vi "Set Version Number.vi"(8 "error in (no error)":errorcluster, 10 "Version number":T1, 11 "NI_AB_API_Targetfile in":refnum<class "NI_AB_API_Build.lvclass">) -> (0 "error out":errorcluster, 3 "NI_AB_API_Targetfile out":refnum<class "NI_AB_API_Build.lvclass">)   [LabVIEW 2020, in "NI_AB_API_Build.lvclass"]
uses:
  <vilib>/AppBuilder/AB_API/Build/NI_AB_API_Build.lvclass
  <vilib>/AppBuilder/AB_API/common/AB_API Version Number.ctl
  <vilib>/AppBuilder/AB_API/Build/NI_AB_API_Build.lvclass/NI_AB_API_Build.ctl
  <vilib>/AppBuilder/AB_Classes/Build/AB_Build.lvclass
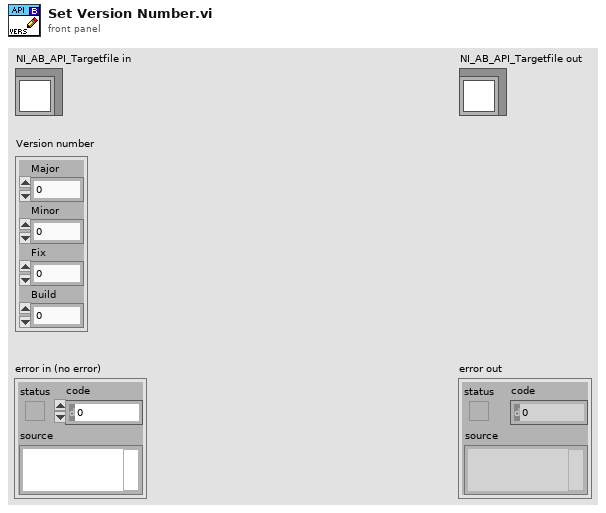
[diagram p1: front panel]
types:
  T1 = typedef "AB_API Version Number.ctl" = cluster{"Major":u16, "Minor":u16, "Fix":u16, "Build":u16}
  T2 = typedef "AB_Build.ctl" = cluster{"buildSpecName":string, "buildSpecDescription":string, "destinations":refnum<class "AB_Destination.lvclass">[], "exclusionOption":T3, "defaultLanguage":string, "supportedLanguages":string[], "excludedDirectories":path[], "buildContext":refnum<vi>, "buildObject":T4, "preview":bool, "programatic":bool, "progressBarEvents":T5, "userLog_Path":path, "preActionID":string, "preAction_Path":path, "postActionID":string, "postAction_Path":path, "eng_checkForBrokenVIs?":bool, "eng_verboseLinkerErrors?":bool, "localDest_Path":path, "targetDest_Path":path, "removeVIObject":u16, "cache":refnum<class "PreviewCache.lvclass">, "use cache":bool, "previewCache_ID":string, "buildCache_ID":string, "eng_TempLocalDest_Path":path, "eng_collectDependencies?":bool, "versionInfo":cluster{"buildVersion":cluster{"major":u16, "minor":u16, "patch":u16, "build":u16}, "autoIncrement":bool}, "eng_enableVIChecksums":bool}
  T3 = typedef "AB_Exclusion_Option.ctl" = cluster{"typedefs":bool, "polymorphicVIs":bool, "unusedLibraryItems":bool, "modifyLibraryFile":bool, "edit-timeDependencies":bool, "inlineVIs":bool, "dependent PPLs":bool, "dependent DLLs":bool}
  T4 = typedef "ItemRef.ctl" = u64
  T5 = typedef "provcom_ProgressBar_Events.ctl" = cluster{"newJob":refnum<user-event>, "newItem":refnum<user-event>, "errorMsg":T6, "cancel":refnum<user-event>}
  T6 = typedef "mxLvBuildError.ctl" = refnum<user-event>
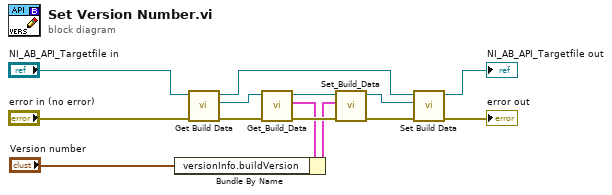
[diagram p0: block diagram]
diagram:
  n1 = call <vilib>:"Get Build Data.vi"("error in (no error)"="error in (no error)", "NI_AB_API_Build in"="NI_AB_API_Targetfile in") -> ("error out"=w2:errorcluster, "AB_Build.lvclass"=w3:refnum<class "AB_Build.lvclass">, "NI_AB_API_Build out"=w6:refnum<class "NI_AB_API_Build.lvclass">)  [unwired: 7 in]
  n2 = call <vilib>:"Get_Build_Data.vi"("error in (no error)"=w2, "Class in"=w3) -> ("error out"=w10:errorcluster, "data"=w8:T2, "Class out"=w9:refnum<class "AB_Build.lvclass">)  [unwired: 7 in]
  n3 = Bundle By Name(cluster=w8, "versionInfo.buildVersion"="Version number") -> (w7:T2)
  n4 = call <vilib>:"Set_Build_Data.vi"("error in (no error)"=w10, "data"=w7, "Class in"=w9) -> ("error out"=w4:errorcluster, "Class out"=w5:refnum<class "AB_Build.lvclass">)  [unwired: 7 in]
  n5 = call <vilib>:"Set Build Data.vi"("error in (no error)"=w4, "AB_Build.lvclass"=w5, "NI_AB_API_Build in"=w6) -> ("error out"=→"error out":errorcluster, "NI_AB_API_Build out"=→"NI_AB_API_Targetfile out":refnum<class "NI_AB_API_Build.lvclass">)  [unwired: 7 in]
